vi "convert_string_to_boolean.vi"(4 "String in":string) -> (1 "boolean value out":bool)   [LabVIEW 2014, in "rszvl_rsidr_core.lvlib"]
uses:
  rszvl_rsidr_core.lvlib
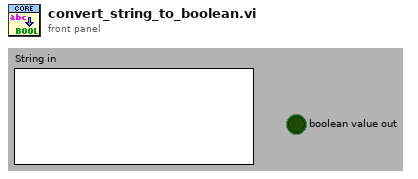
[diagram p1: front panel]
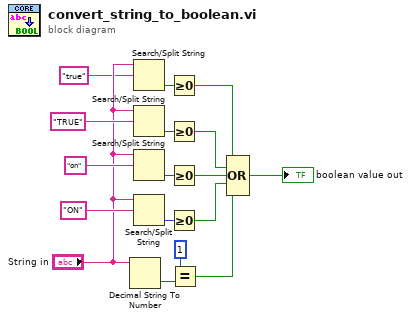
[diagram p0: block diagram]
diagram:
  n1 = Decimal String To Number(string="String in") -> (number=w14:i32)  [unwired: 2 in, 1 out]
  n2 = Search/Split String(string="String in", search string/char (-)="true") -> (offset of match=w2:i32)  [unwired: 1 in, 2 out]
  n3 = Search/Split String(string="String in", search string/char (-)="TRUE") -> (offset of match=w6:i32)  [unwired: 1 in, 2 out]
  n4 = Search/Split String(string="String in", search string/char (-)="on") -> (offset of match=w13:i32)  [unwired: 1 in, 2 out]
  n5 = Search/Split String(string="String in", search string/char (-)="ON") -> (offset of match=w16:i32)  [unwired: 1 in, 2 out]
  n6 = Greater Or Equal To 0?(x=w2) -> (x >= 0?=w1:bool)
  n7 = Greater Or Equal To 0?(x=w6) -> (x >= 0?=w5:bool)
  n8 = Greater Or Equal To 0?(x=w13) -> (x >= 0?=w10:bool)
  n9 = Greater Or Equal To 0?(x=w16) -> (x >= 0?=w9:bool)
  n10 = Equal?(x=1, y=w14) -> (x = y?=w8:bool)
  n11 = Compound Arithmetic op=OR(w1, w5, w10, w9, w8) -> (→"boolean value out":bool)
